vi "FF_SetForce.vi"(7 "Enum":enum16{"Linear", "Bell"}(ring)=enum."Bell", 8 "error in (no error)":errorcluster, 9 "TND":T1, 10 "AnkleVelocity":dbl[](array[numeric]), 11 "Force Field Controller in":refnum<class "ForceField.lvclass">) -> (0 "error out":errorcluster, 1 "ForceNTD":dbl[](array[numeric]), 2 "ForceXYZ":dbl[](array[numeric]), 3 "Force Field Controller out":refnum<class "ForceField.lvclass">)   [LabVIEW 2015, in "ForceField.lvclass"]
uses:
  ForceField.lvclass
  TypeDef/TND.ctl
  ForceField.lvclass/ForceField.ctl
  <vilib>/Analysis/_algsub.llb/Real Vector Norm.vi
  <vilib>/Analysis/baseanly.llb/Real Dot Product.vi
  <vilib>/Analysis/NI_AALPro.lvlib
  <vilib>/Analysis/NI_AALBase.lvlib
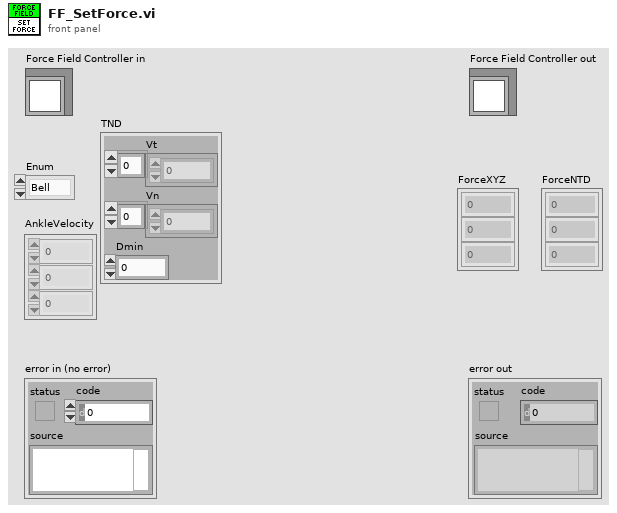
[diagram p1: front panel]
types:
  T1 = typedef "ForceField.lvclass/TND.ctl" = cluster{"Vt":dbl[], "Vn":dbl[], "Dmin":dbl}
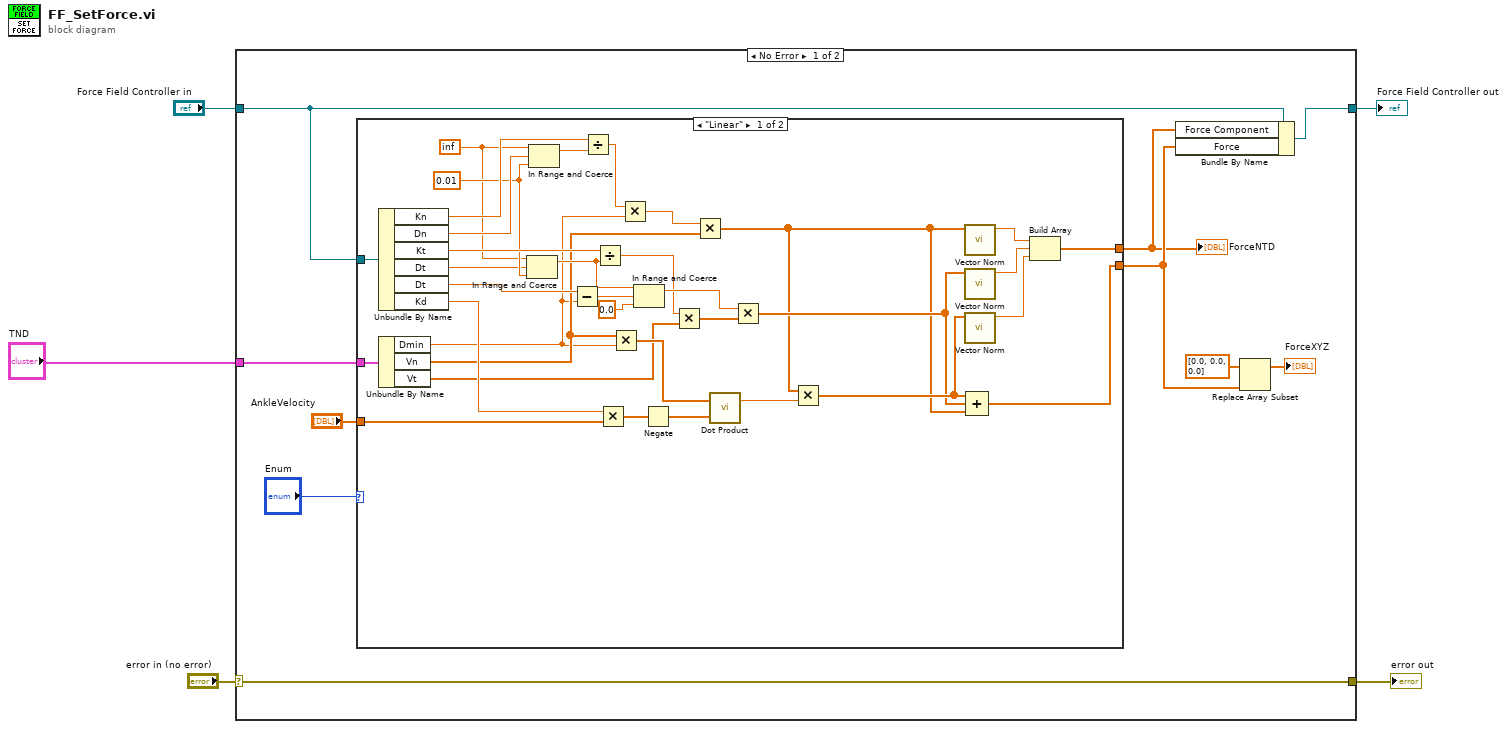
[diagram p0: block diagram]
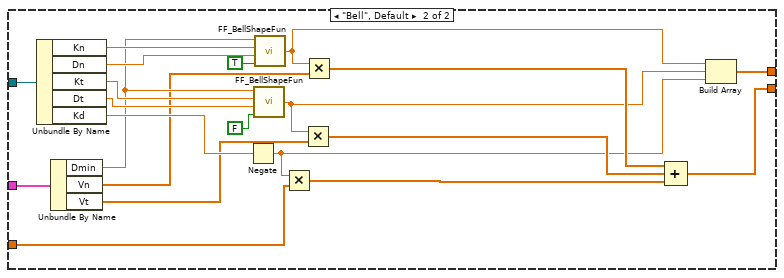
[diagram p2: hidden frame]
diagram:
  n1 = case shown="No Error" "error in (no error)" {
    selector: "error in (no error)" -> [w15 w73]
    tunnel: [w15 w73] -> w4
    tunnel: [w13 w72] -> w2
    tunnel: "Force Field Controller in" -> [w14 w72]
    tunnel: "TND" -> [w6 _]
    frame No Error {
      n2 = case shown="\"Linear\"" "Enum" {
        tunnel: [w50 w64] -> w7
        tunnel: w14 -> [w49 w71]
        tunnel: [w22 w69] -> w8
        tunnel: "AnkleVelocity" -> [w48 w65]
        tunnel: w6 -> [w19 w54]
        frame "Linear" {
          w29 = inf
          w30 = 0.01 ("upper limit")
          n3 = Unbundle By Name(w49) -> ("Kn"=w36:dbl, "Dn"=w33:dbl, "Kt"=w35:dbl, "Dt"=w21:dbl, "Dt"=w20:dbl, "Kd"=w26:dbl)
          n4 = Unbundle By Name(w19) -> ("Dmin"=w16:dbl, "Vn"=w17:dbl[], "Vt"=w18:dbl[])
          n5 = In Range and Coerce(upper limit=w29, x=w21, lower limit=w30) -> (coerced(x)=w31:dbl)  [unwired: 1 out]
          n6 = In Range and Coerce(upper limit=w29, x=w33, lower limit=w30) -> (coerced(x)=w32:dbl)  [unwired: 1 out]
          n7 = Subtract(x=w20, y=w16) -> (x-y=w39:dbl)
          n8 = Divide(x=w36, y=w32) -> (x/y=w28:dbl)
          n9 = Divide(x=w35, y=w31) -> (x/y=w34:dbl)
          n10 = Multiply ("Multiply.vi")(x=w26, y=w48) -> (x*y=w44:dbl[])
          n11 = Multiply(x=w17, y=w16) -> (x*y=w43:dbl[])
          n12 = Multiply(x=w28, y=w16) -> (x*y=w27:dbl)
          n13 = In Range and Coerce(upper limit=w31, x=w39, lower limit=0.0) -> (coerced(x)=w37:dbl)  [unwired: 1 out]
          n14 = Negate(x=w44) -> (-x=w42:dbl[])
          n15 = Multiply(x=w34, y=w18) -> (x*y=w40:dbl[])
          n16 = Multiply(x=w27, y=w17) -> (x*y=w23:dbl[])
          n17 = call-poly <vilib>:"Dot Product.vi"("Y Vector"=w42, "X Vector"=w43) -> ("X * Y"=w41:dbl)  [unwired: 1 out]
          n18 = Multiply(x=w37, y=w40) -> (x*y=w24:dbl[])
          n19 = Multiply(x=w23, y=w41) -> (x*y=w25:dbl[])
          n20 = call-poly <vilib>:"Vector Norm.vi"("Input Vector"=w23) -> ("norm"=w45:dbl)  [unwired: 9 in, 1 out]
          n21 = call-poly <vilib>:"Vector Norm.vi"("Input Vector"=w24) -> ("norm"=w46:dbl)  [unwired: 9 in, 1 out]
          n22 = call-poly <vilib>:"Vector Norm.vi"("Input Vector"=w25) -> ("norm"=w47:dbl)  [unwired: 9 in, 1 out]
          n23 = Compound Arithmetic op=ADD(w25, w24, w23) -> (w22:dbl[])
          n24 = Build Array(w45, w46, w47) -> (w50:dbl[])
        }
        frame "Bell", Default {
          n25 = Unbundle By Name(w71) -> ("Kn"=w63:dbl, "Dn"=w62:dbl, "Kt"=w61:dbl, "Dt"=w60:dbl, "Kd"=w70:dbl)
          n26 = Unbundle By Name(w54) -> ("Dmin"=w53:dbl, "Vn"=w51:dbl[], "Vt"=w52:dbl[])
          n27 = Negate(x=w70) -> (-x=w55:dbl)
          n28 = call "FF_BellShapeFun.vi"("Invert(F)"=FALSE ("Invert"), "(r)adius"=w60, "(A)mplitude"=w61, "x"=w53) -> ("y"=w56:dbl)  [unwired: 2 in]
          n29 = call "FF_BellShapeFun.vi"("Invert(F)"=TRUE ("Invert"), "(r)adius"=w62, "(A)mplitude"=w63, "x"=w53) -> ("y"=w57:dbl)  [unwired: 2 in]
          n30 = Multiply(x=w55, y=w65) -> (x*y=w66:dbl[])
          n31 = Multiply(x=w56, y=w52) -> (x*y=w67:dbl[])
          n32 = Multiply(x=w57, y=w51) -> (x*y=w68:dbl[])
          n33 = Compound Arithmetic op=ADD(w68, w67, w66) -> (w69:dbl[])
          n34 = Build Array(w57, w56, w55) -> (w64:dbl[])
        }
      }
      "ForceNTD" <- w7
      n35 = Bundle By Name(cluster=w14, "Force Component"=w7, "Force"=w8) -> (w13:refnum<class "ForceField.lvclass">)
      n36 = Replace Array Subset(array=dbl[] [0.0, 0.0, 0.0], new element=w8) -> (→"ForceXYZ":dbl[])  [unwired: 1 in]
    }
    frame Error {
    }
  }
  "error out" <- w4
  "Force Field Controller out" <- w2
